vi "Symeetry.vi"() -> ()   [LabVIEW 2014]
doc: "Use this template to build a VI to use as a subVI."
uses:
  <vilib>/vision/NI_Vision_Development_Module.lvlib
panel:
  out "Src":T1(plugin-control)
  out "Dst":T1(plugin-control)
  # ":: MVi Framework V1.0 ::\nAuthor:Gaoke Yang\nEmail: gaoke.yang@yahoo.com\nWeb: www.mvicontrol.com\nCopyright (C) 2015, MVI Technologies All Rights Reserved"
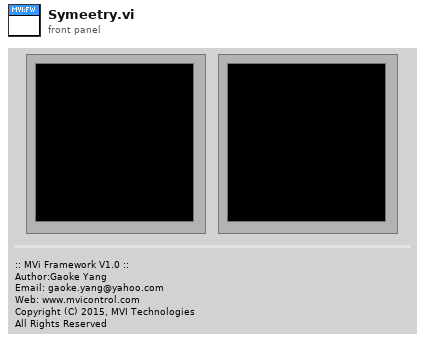
[diagram p1: front panel]
types:
  T1 = typedef "IMAQ Image.ctl" = refnum<image>
  T2 = typedef "Image Type" = u32
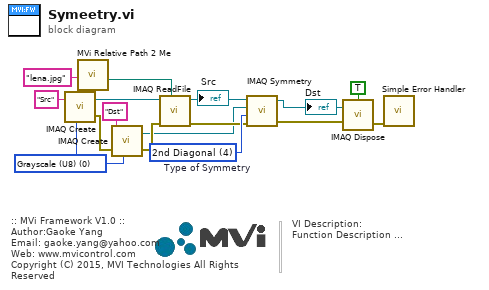
[diagram p0: block diagram]
diagram:
  w6 = u32 4 items=["Horizontal", "Vertical", "Central", "1st Diagonal", "2nd Diagonal"]  # Type of Symmetry
  w10 = T2 0 items=["Grayscale (U8)", "Grayscale (I16)", "Grayscale (SGL)", "Complex (CSG)", "RGB (U32)", "HSL (U32)", "RGB (U64)", "Grayscale (U16)"] ("Image Type")
  # "VI Description:\nFunction Description ..."
  # ":: MVi Framework V1.0 ::\nAuthor:Gaoke Yang\nEmail: gaoke.yang@yahoo.com\nWeb: www.mvicontrol.com\nCopyright (C) 2015, MVI Technologies All Rights Reserved"
  n1 = call "IMAQ Create"("Image Name"="Src" ("name or relative path"), "Image Type"=w10) -> ("New Image"=w7:T1, "error out"=w9:errorcluster)  [unwired: 2 in, 1 out]
  n2 = call "MVi Relative Path 2 Me.vi"("Relative Path"="lena.jpg" ("name or relative path")) -> ("Appended Dir"=w12:path)  [unwired: 5 in, 1 out]
  n3 = call "IMAQ Create"("Image Name"="Dst" ("name or relative path"), "Image Type"=w10, "error in (no error)"=w9) -> ("New Image"=w3:T1, "error out"=w8:errorcluster)  [unwired: 1 in, 1 out]
  n4 = call "IMAQ ReadFile"("File Path"=w12, "error in (no error)"=w8, "Image"=w7) -> ("error out"=w5:errorcluster, "Image Out"=w1:T1)  [unwired: 4 in, 3 out]
  "Src" <- w1
  n5 = call "IMAQ Symmetry"("error in (no error)"=w5, "Type of Symmetry"=w6, "Image Dst"=w3, "Image Src"=w1) -> ("error out"=w4:errorcluster, "Image Dst Out"=w2:T1)  [unwired: 1 in]
  "Dst" <- w2
  n6 = call "IMAQ Dispose"("All Images? (No)"=TRUE, "Image"=w2, "error in (no error)"=w4) -> ("error out"=w13:errorcluster)  [unwired: 3 out]
  n7 = call <vilib>:"Simple Error Handler.vi"("error in (no error)"=w13) -> ()  [unwired: 1 in, 8 out]
